vi "to_celsius_sub.vi"(11 "Bytes Read":u8[](array[numeric])) -> (3 "Numeric":dbl)   [LabVIEW 2021]
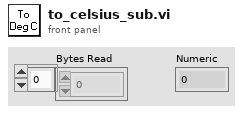
[diagram p1: front panel]
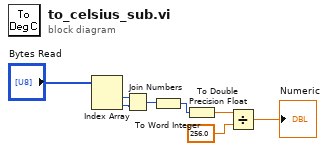
[diagram p0: block diagram]
diagram:
  n1 = Index Array(array="Bytes Read") -> (element #1=w2:u8, element #2=w3:u8)  [unwired: 2 in]
  n2 = Join Numbers(hi=w2, lo=w3) -> ((hi.lo)=w1:u16)
  n3 = To Word Integer(number=w1) -> (16bit integer=w8:i16)
  n4 = To Double Precision Float(number=w8) -> (double precision float=w7:dbl)
  n5 = Divide(x=w7, y=256.0) -> (x/y=→"Numeric":dbl)
